vi "readCommand.vi"(8 "error in (no error)":errorcluster, 11 "InternalCommandId in":refnum<class "InternalCommandId.lvclass">) -> (0 "error out":errorcluster, 1 "CommandValue":T1, 2 "CommandID":i32, 3 "InternalCommandId out":refnum<class "InternalCommandId.lvclass">)   [LabVIEW 2016, in "InternalCommandId.lvclass"]
uses:
  InternalCommandId.lvclass
  ts_electrometeruserevents/Typedefs/CommandValue.ctl
  ts_electrometeruserevents/Typedefs/ElectrometerTypedefs.lvlib
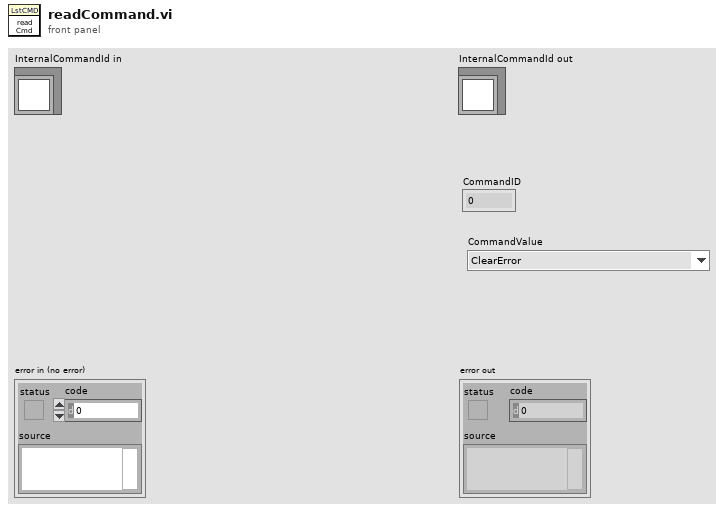
[diagram p1: front panel]
types:
  T1 = typedef "ElectrometerTypedefs.lvlib/CommandValue.ctl" = enum16{"ClearError", "Disable", "Enable", "Exit", "GoToStandby", "OnHeartbeat", "OnIncomingMessagingError", "OnInterrupt", "Start", "SetDigitalFilter", "StartScan", "StartScanDt", "StartScanReachIntensity", "StopScan", "SetIntegrationTime", "PerformZeroCalib", "SetRange", "SetMode", "Power"}
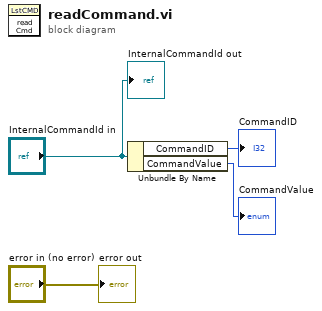
[diagram p0: block diagram]
diagram:
  n1 = Unbundle By Name("InternalCommandId in") -> ("CommandID"=→"CommandID":i32, "CommandValue"=→"CommandValue":T1)
  "error out" <- "error in (no error)"
  "InternalCommandId out" <- "InternalCommandId in"
